vi "Parse.vi"(8 "Error In":errorcluster, 11 "object in":refnum<class "2021_2.lvclass">) -> (0 "Error Out":errorcluster, 3 "object out":refnum<class "2021_2.lvclass">)   [LabVIEW 2020, in "2021_2.lvclass"]
uses:
  2021_2.lvclass
  2021_2.lvclass/2021_2.ctl
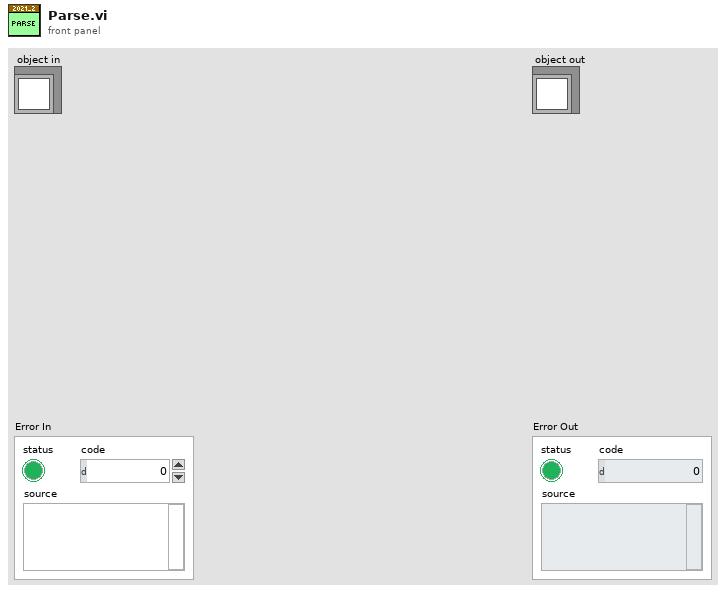
[diagram p1: front panel]
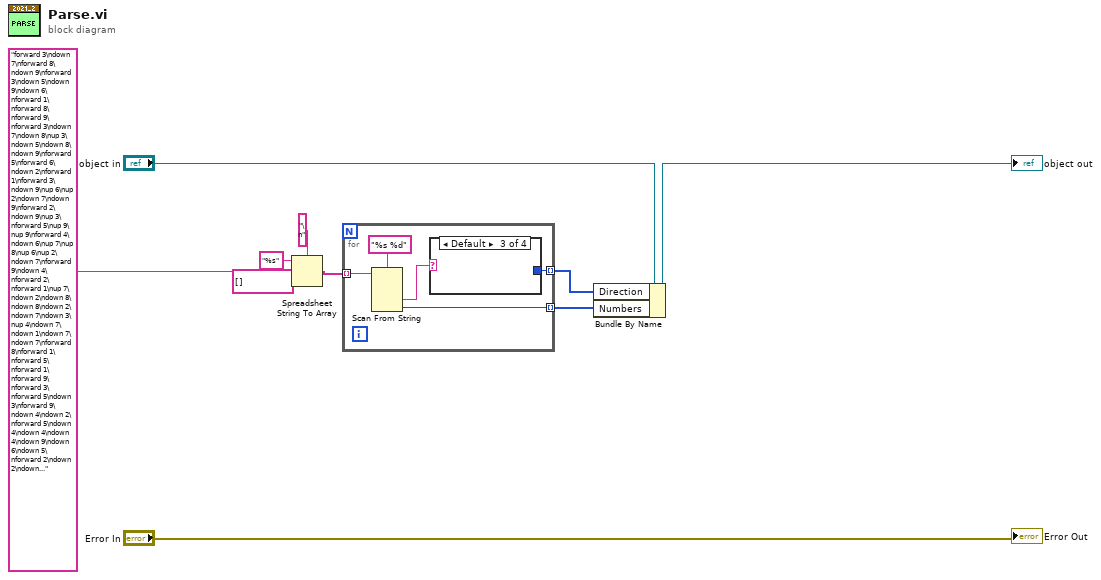
[diagram p0: block diagram]
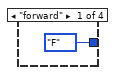
[diagram p2: hidden frame]
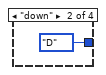
[diagram p3: hidden frame]
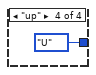
[diagram p4: hidden frame]
diagram:
  n1 = Spreadsheet String To Array(delimiter (Tab)="\n", format string="%s", spreadsheet string="forward 3\ndown 7\nforward 8\ndown 9\nforward 3\ndown 5\ndown 9\ndown 6\nforward 1\nforward 8\nforward 9\nforward 3\ndown 7\ndown 8\nup 3\ndown 5\ndown 8\ndown 9\nforward 5\nforward 6\ndown 2\nforward 1\nforward 3\ndown 9\nup 6\nup 2\ndown 7\ndown 9\nforward 2\ndown 9\nup 3\nforward 5\nup 9\nup 9\nforward 4\ndown 6\nup 7\nup 8\nup 6\nup 2\ndown 7\nforward 9\ndown 4\nforward 2\nforward 1\nup 7\ndown 2\ndown 8\ndown 8\ndown 2\ndown 7\ndown 3\nup 4\ndown 7\ndown 1\ndown 7\ndown 7\nforward 8\nforward 1\nforward 5\nforward 1\nforward 9\nforward 3\nforward 5\ndown 3\nforward 9\ndown 4\ndown 2\nforward 5\ndown 4\ndown 4\ndown 4\ndown 9\ndown 6\ndown 5\nforward 2\ndown 2\ndown 8\ndown 8\ndown 7\ndown 2\ndown 8\ndown 6\ndown 4\ndown 7\nup 8\nup 7\nup 6\ndown 4\ndown 2\nup 4\nup 8\nup 4\ndown 4\ndown 3\nforward 7\nforward 8\nup 1\nup 1\nup 7\nforward 2\ndown 2\nforward 7\nforward 7\nforward 7\ndown 2\ndown 2\nforward 5\ndown 3\nforward 3\ndown 6\ndown 9\ndown 4\ndown 1\nforward 2\nforward 2\ndown 8\ndown 9\nup 3\nforward 8\ndown 7\nforward 6\nforward 6\ndown 9\nup 2\nup 9\ndown 2\ndown 8\nup 2\nforward 6\ndown 5\nup 9\nforward 6\ndown 3\ndown 9\nforward 8\nforward 8\nforward 1\nforward 6\ndown 7\nforward 3\nforward 5\nforward 6\ndown 1\ndown 1\nforward 3\nforward 8\nforward 8\nup 5\ndown 6\nup 5\ndown 1\nup 3\ndown 6\nforward 1\nup 3\nup 4\ndown 8\ndown 2\nup 2\nforward 1\nforward 2\nforward 6\nup 2\ndown 3\nup 5\ndown 5\ndown 7\nup 6\nup 6\ndown 8\nforward 7\nforward 2\nforward 3\nup 5\ndown 5\ndown 6\ndown 4\nforward 8\nup 1\nforward 5\nup 1\nforward 4\nforward 3\nforward 4\ndown 2\nup 5\nup 4\ndown 5\nforward 1\nforward 8\ndown 7\ndown 1\ndown 7\nforward 6\ndown 4\ndown 6\nforward 6\ndown 8\nforward 7\ndown 4\ndown 8\nup 7\ndown 6\ndown 2\nup 8\ndown 7\ndown 8\ndown 6\ndown 3\nup 1\ndown 7\nforward 1\ndown 3\ndown 5\ndown 9\ndown 3\nforward 1\nforward 4\nforward 2\ndown 8\nforward 7\ndown 3\ndown 7\nforward 7\ndown 4\ndown 5\ndown 1\nforward 2\ndown 7\nforward 3\nforward 4\ndown 8\nup 6\ndown 4\nup 5\nforward 5\nforward 7\nup 8\nforward 6\nup 3\nforward 9\nup 9\ndown 1\ndown 2\nforward 6\ndown 5\nforward 6\ndown 7\nforward 9\ndown 2\nup 5\ndown 2\nforward 3\nup 7\nforward 3\ndown 4\nforward 7\nforward 8\ndown 5\nup 7\nup 8\nforward 7\ndown 4\nforward 9\nforward 6\ndown 2\nforward 3\nup 8\nup 4\nforward 2\nforward 4\nforward 1\ndown 6\nforward 1\ndown 9\nforward 2\nup 5\ndown 2\ndown 5\ndown 5\ndown 2\ndown 9\ndown 4\nforward 5\ndown 5\nup 1\nforward 4\ndown 6\ndown 5\nup 8\nup 4\ndown 8\nforward 4\ndown 8\nforward 4\ndown 2\ndown 8\nforward 3\nforward 7\ndown 1\nforward 3\nforward 7\nforward 1\ndown 4\nforward 2\ndown 3\ndown 4\nforward 1\nup 6\nforward 8\ndown 5\nup 6\nup 3\nforward 7\ndown 3\nforward 4\nforward 9\nforward 2\nup 2\nup 7\nforward 1\nup 8\ndown 6\nup 5\ndown 3\nup 7\ndown 4\nup 7\ndown 8\ndown 7\nforward 5\nup 7\ndown 1\nup 9\ndown 2\ndown 8\ndown 5\nforward 4\ndown 3\nup 4\ndown 2\nforward 6\ndown 2\nforward 9\nup 9\nup 8\nforward 3\nforward 7\nforward 7\nup 4\nup 3\nup 4\nforward 1\ndown 2\nup 6\ndown 2\ndown 4\nup 3\ndown 8\ndown 9\ndown 4\nforward 6\ndown 5\ndown 5\nforward 7\ndown 2\nforward 8\nup 2\nup 7\ndown 5\ndown 7\nup 9\nup 4\nup 5\ndown 4\ndown 8\ndown 9\ndown 7\ndown 1\ndown 1\nup 7\nup 8\ndown 5\nforward 2\nup 3\ndown 2\ndown 9\ndown 4\nforward 1\nforward 1\nup 4\ndown 9\nup 7\nforward 7\nup 8\nup 4\ndown 2\ndown 1\nforward 2\nup 4\ndown 3\nup 7\ndown 7\ndown 6\ndown 4\nup 3\ndown 7\nforward 5\ndown 6\ndown 9\ndown 3\nforward 1\ndown 6\nforward 3\ndown 5\nup 1\nforward 5\nforward 4\nforward 8\nforward 1\nup 4\ndown 2\ndown 7\ndown 9\nup 4\nup 6\nforward 8\nup 4\ndown 8\nforward 7\nforward 1\ndown 7\nforward 9\nforward 1\nforward 7\nforward 9\ndown 3\nforward 4\ndown 3\ndown 3\ndown 3\ndown 1\ndown 5\nforward 1\nforward 7\nup 5\nforward 5\nforward 4\nforward 7\ndown 7\nup 5\nforward 1\nforward 8\ndown 3\nup 6\ndown 7\nforward 6\ndown 8\nforward 6\nup 4\ndown 9\nup 1\nforward 4\nforward 8\ndown 5\nforward 7\nup 9\nforward 2\nup 2\nforward 7\ndown 3\nforward 2\ndown 7\ndown 1\nforward 9\nforward 3\nup 5\nforward 7\nup 4\nforward 2\ndown 3\ndown 2\ndown 8\nforward 7\ndown 8\ndown 3\nforward 9\nforward 9\nforward 5\nup 8\nforward 9\nup 2\nforward 2\nup 4\nforward 2\nforward 1\nforward 7\nforward 6\ndown 5\nforward 5\nforward 1\nforward 7\nforward 4\ndown 5\ndown 9\ndown 8\nforward 5\nup 5\nup 1\ndown 8\ndown 9\nforward 1\ndown 5\nforward 6\ndown 1\ndown 7\ndown 7\ndown 4\nforward 3\ndown 5\ndown 8\nforward 2\ndown 4\nforward 3\ndown 1\nup 5\ndown 8\nforward 9\nup 6\nup 4\ndown 6\ndown 9\nforward 2\nforward 5\ndown 3\nforward 2\ndown 5\nforward 1\nforward 4\ndown 6\ndown 4\nup 2\ndown 9\nforward 2\nup 8\ndown 4\nforward 7\ndown 5\nforward 8\ndown 1\nforward 5\ndown 7\nup 5\ndown 7\ndown 4\nforward 3\ndown 1\nforward 7\nforward 9\nup 9\nforward 5\nforward 8\nup 8\nforward 6\ndown 5\ndown 8\nforward 9\nforward 3\ndown 3\nforward 9\nforward 7\nforward 6\nforward 1\nup 2\nforward 8\ndown 9\ndown 5\ndown 5\ndown 4\nforward 7\ndown 8\ndown 7\nforward 8\nforward 2\ndown 5\nforward 2\nforward 3\ndown 6\ndown 8\nup 8\nforward 7\ndown 7\nup 7\nforward 5\nup 6\nforward 7\nup 6\nforward 8\nforward 5\nup 6\nforward 1\ndown 5\nforward 1\nup 5\ndown 1\nforward 6\nforward 3\nup 2\nforward 9\nforward 8\ndown 9\nforward 7\nforward 7\nforward 8\nup 9\ndown 8\nup 1\ndown 4\nforward 2\nforward 7\ndown 1\nup 7\ndown 5\nforward 2\ndown 4\ndown 8\nforward 6\ndown 3\nforward 8\nup 6\nforward 5\nforward 7\ndown 5\ndown 1\ndown 7\ndown 7\nup 8\ndown 5\nforward 4\ndown 5\ndown 7\ndown 2\nup 8\nforward 6\nup 1\ndown 3\nforward 9\nup 1\ndown 7\nforward 2\ndown 6\nforward 6\nup 3\nup 9\nup 2\nforward 4\nforward 4\ndown 4\ndown 4\ndown 2\ndown 5\nforward 7\nforward 6\nforward 9\ndown 9\nforward 6\nup 1\ndown 2\ndown 4\ndown 7\ndown 5\ndown 4\nup 2\nup 8\ndown 6\nforward 2\nup 7\ndown 2\nup 5\ndown 8\nforward 3\nup 2\nforward 3\nforward 5\nforward 9\nforward 2\nforward 8\nforward 1\ndown 5\nup 6\nforward 9\nforward 4\nup 8\ndown 8\nup 2\ndown 9\ndown 3\ndown 5\nup 4\nforward 2\ndown 5\nforward 6\ndown 6\nforward 2\nforward 7\nforward 6\nforward 1\ndown 7\nforward 8\nup 2\nforward 5\nforward 5\nup 3\nforward 2\nforward 3\nforward 8\nforward 4\ndown 1\ndown 9\nup 5\ndown 5\nforward 1\ndown 8\nup 3\ndown 9\nforward 5\nforward 2\nforward 2\nup 1\nforward 1\ndown 5\nforward 4\nup 4\nup 3\nup 3\ndown 4\ndown 5\ndown 1\nforward 8\ndown 4\nup 7\ndown 6\nforward 5\nforward 4\nforward 8\nforward 8\nup 3\nforward 7\ndown 4\nforward 8\nforward 4\nforward 6\ndown 8\ndown 6\ndown 1\nforward 4\ndown 8\ndown 6\nforward 2\ndown 8\nup 7\ndown 2\nforward 5\ndown 4\ndown 7\ndown 8\nforward 5\ndown 4\ndown 2\ndown 7\ndown 4\nforward 7\nforward 3\nup 4\ndown 7\ndown 9\nup 4\nup 5\ndown 7\nup 5\ndown 3\ndown 5\nforward 8\nup 1\nup 9\nforward 9\nforward 7\ndown 2\nup 1\nup 7\ndown 3\nforward 3\nup 6\nforward 1\nforward 2\ndown 4\ndown 3\nforward 4\nforward 7\nforward 9\ndown 8\ndown 6\nforward 1\nforward 3\nforward 2\nup 3\ndown 6\ndown 7\nup 8\ndown 5\nup 6\ndown 8\nforward 4\nup 3\nforward 3\nforward 4\ndown 5\nup 5\ndown 4\ndown 5\ndown 5\nforward 3\nup 9\ndown 8\ndown 2\ndown 7\ndown 4\ndown 3\nup 2\nforward 6\ndown 4\ndown 1\ndown 4\nforward 1\nforward 8\ndown 3\ndown 7\ndown 3\nforward 1\ndown 9\ndown 7\ndown 3\ndown 3\ndown 6\ndown 8\ndown 2\ndown 5\nup 1\nup 7\nforward 9\nforward 6\nforward 7\nforward 8\nup 7\ndown 9\ndown 4\ndown 7\nforward 2\nforward 4\nforward 1\nforward 4\nforward 3\nforward 8\ndown 5\nforward 8\nup 4\nup 9\nforward 3\ndown 7\nforward 9\ndown 2\nforward 5\nup 7\ndown 4\ndown 3\ndown 5\ndown 4\nforward 9\nforward 5\nforward 6\nforward 6\ndown 2\ndown 7\nforward 4\nup 5\ndown 8\ndown 9\nforward 5\ndown 8\nforward 9\nup 6\nforward 8\nforward 7\nup 7\ndown 9\nforward 5\ndown 9\nforward 7\ndown 5\ndown 7\nforward 9\nforward 4\nup 1\nup 9\nforward 7\nup 5\nup 2\ndown 6\nforward 7\ndown 2\nforward 6\nforward 7\ndown 4\nup 3\nup 9\nforward 4\nforward 6\nforward 3\nup 6\ndown 5\nup 2\nforward 3\ndown 5\nforward 1\nup 7\ndown 8\nup 4\nforward 9\nforward 6\ndown 7\nforward 4\ndown 9\ndown 8\ndown 7\nforward 7\ndown 5\nforward 3\nup 5\nforward 9\nforward 7\nforward 3\ndown 5\nforward 8\ndown 3\nforward 1\ndown 3\ndown 3\nforward 2\ndown 4\nforward 7\nup 1\ndown 6\nup 3\nforward 8\ndown 6\nforward 6\ndown 5\ndown 4\nforward 3\nup 1\nforward 5\nforward 5\nforward 2\nup 9\nforward 3\ndown 5\nup 3\nup 4\ndown 7\ndown 4\nup 3\nup 3\nforward 2\nup 2\nforward 8\ndown 9\ndown 1\nup 8\ndown 2\nup 4\nforward 9\nup 1\ndown 8\nforward 3\nup 9\ndown 7\ndown 5\ndown 9\ndown 1\ndown 2\ndown 9\ndown 4\ndown 8\ndown 8\ndown 9\ndown 2\ndown 6\ndown 9\nforward 8" ("PuzzleInput"), array type (2D Dbl)=string[] []) -> (array=w3:string[])
  n2 = for {
    tunnel: w3 -> [w15] mode=indexing
    tunnel: [w13] -> w2 mode=indexing
    tunnel: [w11] -> w1 mode=indexing
    n3 = Scan From String(format string="%s %d", input string=w15) -> (output 1=w12:string, output 2=w13:i32)  [unwired: 4 in, 3 out]
    n4 = case shown="Default" w12 {
      tunnel: [enum16{"F", "D", "U"}."F" ("Direction") enum16{"F", "D", "U"}."D" ("Direction") _ enum16{"F", "D", "U"}."U" ("Direction")] -> w11
      frame "forward" {
      }
      frame "down" {
      }
      frame Default {
      }
      frame "up" {
      }
    }
  }
  n5 = Bundle By Name(cluster="object in", "Direction"=w1, "Numbers"=w2) -> (→"object out":refnum<class "2021_2.lvclass">)
  "Error Out" <- "Error In"
